vi "getExposureTime.vi"(8 "error in (no error)":errorcluster, 11 "Camera in":refnum<class "Camera.lvclass">) -> (0 "error out":errorcluster, 2 "exposure_time_s":dbl, 3 "Camera out":refnum<class "Camera.lvclass">)   [LabVIEW 2019, in "Camera.lvclass"]
doc: "Sets the exposure time of the camera. The values for the underlying pco.sdk function PCO_SetDelayExposureTime.vi will be calculated automatically. The delay time is set to 0."
uses:
  Camera.lvclass
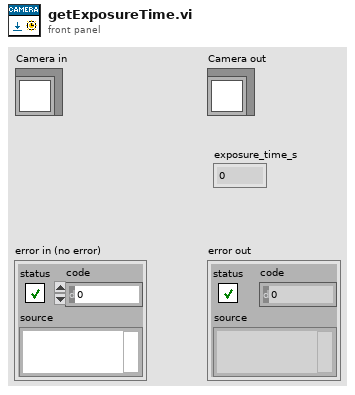
[diagram p1: front panel]
types:
  T1 = typedef "Camera.lvclass/binning.ctl" = cluster{"vert":u16, "horz":u16}
  T2 = cluster{"exposure_time_s":dbl, "delay_time_s":dbl, "roi":cluster{"x0":u64, "y0":u64, "x1":u64, "y1":u64}, "timestamp_mode":u16, "pixelrate":u32, "trigger_mode":u16, "acquire_mode":u16, "metadata_mode":u16, "noisefilter_mode":u16, "binning":T1}
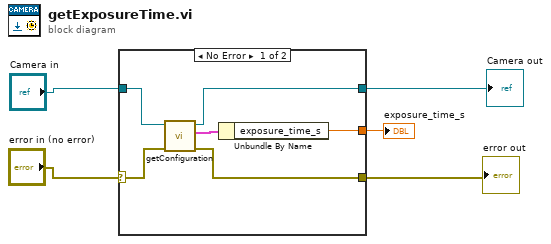
[diagram p0: block diagram]
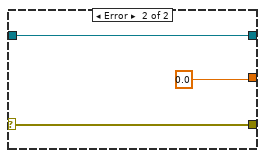
[diagram p2: hidden frame]
diagram:
  n1 = case shown="No Error" "error in (no error)" {
    selector: "error in (no error)" -> [w10 w14]
    tunnel: [w6 w14] -> w5
    tunnel: [w7 w13] -> w4
    tunnel: "Camera in" -> [w11 w13]
    tunnel: [w8 0.0 ("exposure_time_s")] -> w1
    frame No Error {
      n2 = call-dynamic "getConfiguration.vi"("error in (no error)"=w10, "Camera in"=w11) -> ("error out"=w6:errorcluster, "configuration"=w9:T2, "Camera out"=w7:refnum<class "Camera.lvclass">)  [unwired: 7 in]
      n3 = Unbundle By Name(w9) -> ("exposure_time_s"=w8:dbl)
    }
    frame Error {
    }
  }
  "error out" <- w5
  "Camera out" <- w4
  "exposure_time_s" <- w1
